vi "example_01.vi"() -> ()   [LabVIEW 2015, in "lv-recipe-machine.lvlib"]
uses:
  lv-recipe-machine.lvlib
  _controls/example_01_manual_actions.ctl
  public/_controls/step.ctl
  public/_controls/step_vi_reference.ctl
  public/_controls/mode.ctl
  _subvis/manual_test_comparison.vi
  _subvis/manual_test_wait.vi
  lv-recipe-machine_/repub-dvr_nre.lvlib
panel:
  out "data":variant
  in  "stop":bool
  in  "manual_action":T1=enum."test_random"
  in  "execute":bool
  in  "recipe":T2(ring)
  in  "resume":bool
  in  "abort":bool
  in  "pause":bool
  in  "start":bool
  in  "manual_mode":bool
  in  "automatic_mode":bool
  out "wait_elapsed_time":dbl format="%<%H:%M:%S>t"
  out "recipe_elapsed_time":dbl format="%<%H:%M:%S>t"
  out "random_data":dbl
  out "action":string
  out "state":string
  out "mode":string
  in  "events":i32(listbox)
  out "error out":errorcluster
  # "Manual Inputs"
  # "Automatic Inputs"
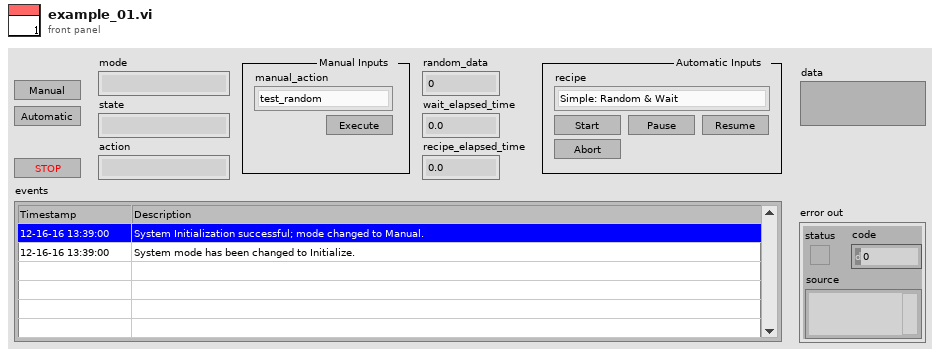
[diagram p1: front panel]
types:
  T1 = typedef "lv-recipe-machine.lvlib/example_01_manual_actions.ctl" = enum16{"<manual_action>", "test_random", "test_comparison", "test_wait", "<null>"}
  T2 = enum16{"Simple: Random & Wait", "Simple: Random & Test", "Intermediate: Fixed Continuous", "Intermediate: Test w/Continuous-Fail"}
  T3 = typedef "lv-recipe-machine.lvlib/step.ctl" = cluster{"name":string, "step_vi_reference":T4, "data":variant}
  T4 = typedef "lv-recipe-machine.lvlib/step_vi_reference.ctl" = refnum<vi>
  T5 = typedef "repub-dvr_nre.lvlib/references.ctl" = cluster{"semaphore":T6, "input_queue":refnum<queue>, "output_queue":refnum<queue>, "data_dvr":refnum<data-value>, "stop_notifier":refnum<notifier>, "transition_queue":refnum<queue>, "change_in_notifier":refnum<notifier>, "change_out_notifier":refnum<notifier>, "change_in_event":refnum<user-event>, "change_out_event":refnum<user-event>}
  T6 = typedef "Semaphore RefNum" = refnum<k1>
  T7 = typedef "lv-recipe-machine.lvlib/mode.ctl" = enum16{"<mode>", "manual", "automatic", "<null>"}
  T8 = typedef "repub-dvr_nre.lvlib/status.ctl" = cluster{"mode":T7, "manual_state":T9, "automatic_state":T10, "step":string}
  T9 = typedef "lv-recipe-machine.lvlib/manual_state.ctl" = enum16{"<manual_state>", "failed", "action", "running", "idle", "<null>"}
  T10 = typedef "lv-recipe-machine.lvlib/automatic_state.ctl" = enum16{"<automatic_state>", "failed", "idle", "running", "paused", "transition", "stopped", "<null>"}
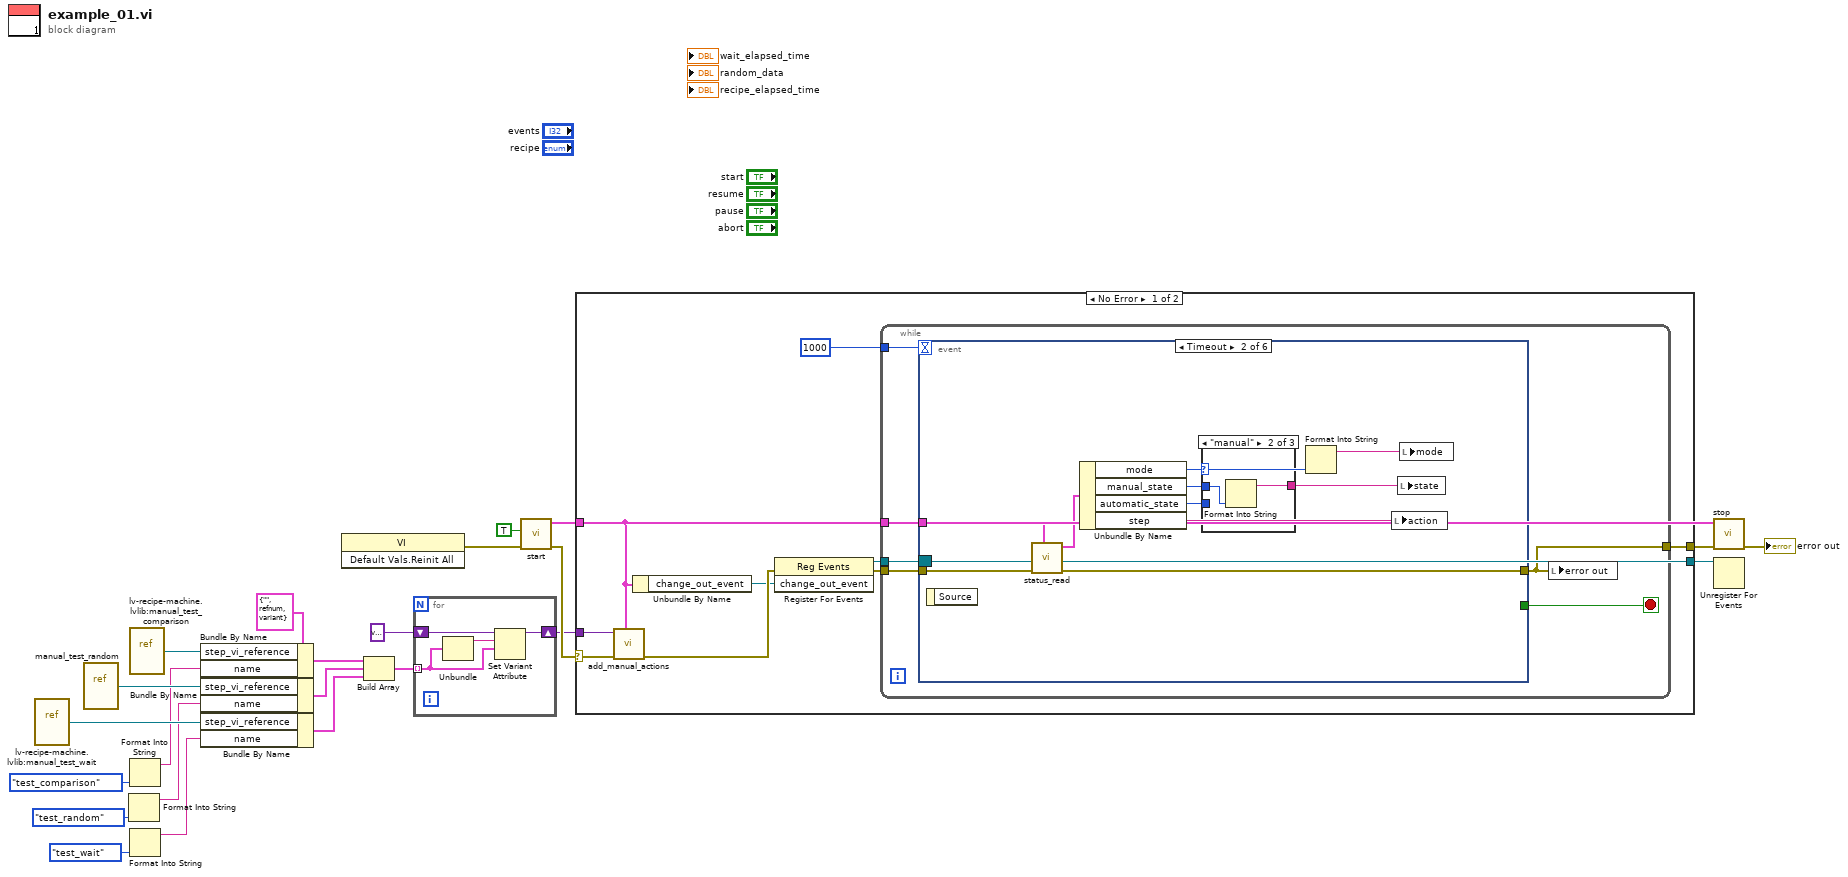
[diagram p0: block diagram]
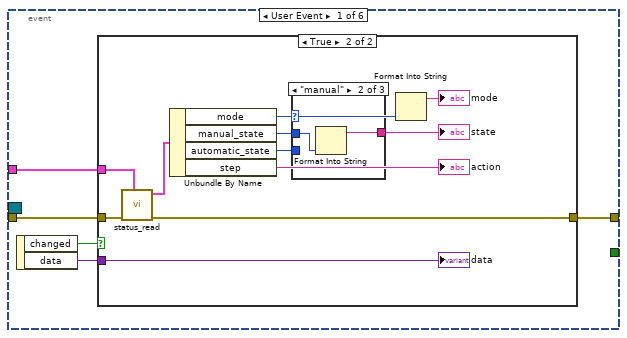
[diagram p2: hidden frame]
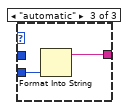
[diagram p5: hidden frame]
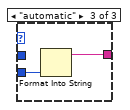
[diagram p7: hidden frame]
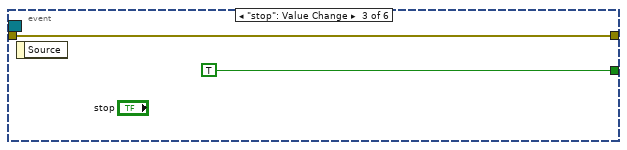
[diagram p8: hidden frame]
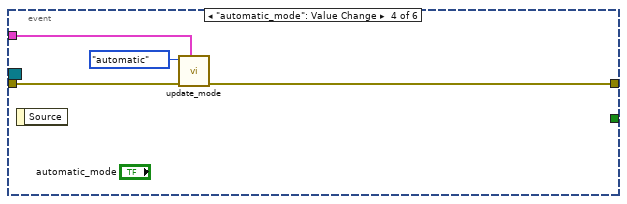
[diagram p9: hidden frame]
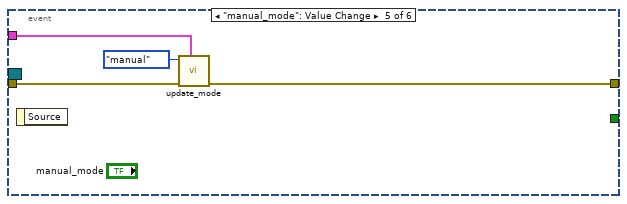
[diagram p10: hidden frame]
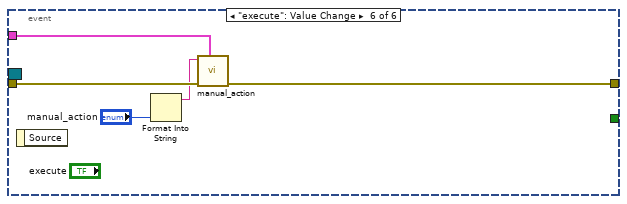
[diagram p11: hidden frame]
diagram:
  w9 = T3 {"name"="", "step_vi_reference"=refnum, "data"=variant} ("step")
  n1 = vi-ref "lv-recipe-machine.lvlib:manual_test_wait.vi"() -> (w4:refnum<vi>)
  n2 = vi-ref "manual_test_random.vi"() -> (w12:refnum<vi>)
  n3 = Format Into String(example_01_manual_actions."test_random" ("action")) -> (resulting string=w2:string)  [unwired: 3 in, 1 out]
  n4 = vi-ref "lv-recipe-machine.lvlib:manual_test_comparison.vi"() -> (w13:refnum<vi>)
  n5 = Format Into String(example_01_manual_actions."test_comparison" ("action")) -> (resulting string=w1:string)  [unwired: 3 in, 1 out]
  n6 = Format Into String(example_01_manual_actions."test_wait" ("action")) -> (resulting string=w3:string)  [unwired: 3 in, 1 out]
  n7 = Bundle By Name(cluster=w9, "step_vi_reference"=w13, "name"=w1) -> (w15:T3)
  n8 = Bundle By Name(cluster=w9, "step_vi_reference"=w12, "name"=w2) -> (w14:T3)
  n9 = Bundle By Name(cluster=w9, "step_vi_reference"=w4, "name"=w3) -> (w8:T3)
  n10 = invoke class="VI" method="Default Vals.Reinit All"() -> (error out=w22:errorcluster)  [unwired: 3 in, 2 out]
  n11 = Build Array(w15, w14, w8) -> (w11:T3[])
  n12 = for {
    tunnel: w11 -> [w25] mode=indexing
    shift-right: [w26] -> w10
    shift-left: variant ("recipe") -> [w27]
    n13 = Unbundle(w25) -> ("name"=w24:string)  [unwired: 2 out]
    n14 = Set Variant Attribute(Variant=w27, name=w24, value=w25) -> (Variant out=w26:variant)  [unwired: 1 in, 2 out]
  }
  n15 = call "start.vi"("error in (no error)"=w22, "enable_event"=TRUE) -> ("error out"=w21:errorcluster, "references"=w20:T5)  [unwired: 8 in]
  n16 = case shown="No Error" w21 {
    selector: w21 -> [w29 w93]
    tunnel: [w35 w93] -> w23
    tunnel: w20 -> [w31 _]
    tunnel: [w32 _] -> w18
    tunnel: w10 -> [w30 _]
    frame No Error {
      n17 = call "add_manual_actions.vi"("references"=w31, "error in (no error)"=w29, "manual_actions"=w30) -> ("error out"=w36:errorcluster)  [unwired: 8 in]
      n18 = Unbundle By Name(w31) -> ("change_out_event"=w33:refnum<user-event>)
      n19 = register-events(error in=w36, w33) -> (reference out=w32:refnum<event-registration>, error out=w34:errorcluster)  [unwired: 1 in]
      n20 = while {
        tunnel: w34 -> [w42]
        tunnel: [w38] -> w35
        tunnel: w31 -> [w40]
        tunnel: w32 -> [w39]
        tunnel: 1000 -> [w37]
        stop <- w41 stop-if-true
        n21 = event shown="[1] Timeout" {
          selector: w39 -> [_ _ _ _ _ _]
          dyn-events: _ -> [_ _ _ _ _ _]
          timeout: w37 -> [_ _ _ _ _ _]
          tunnel: w42 -> [w47 w73 w79 w82 w86 w92]
          tunnel: [w46 w72 w79 w83 w87 w89] -> w38
          tunnel: [_ _ TRUE _ _ _] -> w41
          tunnel: w40 -> [w45 w71 _ w81 w85 w88]
          event User Event {
            n22 = event-data() -> ("changed"=w44:bool, "data"=w43:variant)  [unwired: 1 in]
            n23 = case shown="True" w44 {
              tunnel: w47 -> [w48 w59]
              tunnel: [w48 w56] -> w46
              tunnel: w45 -> [_ w58]
              tunnel: w43 -> [_ w49]
              frame False {
              }
              frame True {
                n24 = call "status_read.vi"("references"=w58, "error in (no error)"=w59) -> ("error out"=w56:errorcluster, "status"=w57:T8)  [unwired: 8 in]
                n25 = Unbundle By Name(w57) -> ("mode"=w53:T7, "manual_state"=w55:T9, "automatic_state"=w54:T10, "step"=→"action":string)
                n26 = case shown="\"manual\"" w53 {
                  tunnel: w55 -> [_ w61 _]
                  tunnel: w54 -> [_ _ w62]
                  tunnel: [_ w60 w63] -> w51
                  frame Default {
                  }
                  frame "manual" {
                    n27 = Format Into String(w61) -> (resulting string=w60:string)  [unwired: 3 in, 1 out]
                  }
                  frame "automatic" {
                    n28 = Format Into String(w62) -> (resulting string=w63:string)  [unwired: 3 in, 1 out]
                  }
                }
                "state" <- w51
                n29 = Format Into String(w53) -> (resulting string=→"mode":string)  [unwired: 3 in, 1 out]
                "data" <- w49
              }
            }
          }
          event Timeout {
            n30 = event-data() -> ()  [unwired: 1 in, 1 out]
            n31 = call "status_read.vi"("references"=w71, "error in (no error)"=w73) -> ("error out"=w72:errorcluster, "status"=w70:T8)  [unwired: 8 in]
            n32 = Unbundle By Name(w70) -> ("mode"=w67:T7, "manual_state"=w69:T9, "automatic_state"=w68:T10, "step"=w64:string)
            n33 = case shown="\"manual\"" w67 {
              tunnel: w69 -> [_ w75 _]
              tunnel: w68 -> [_ _ w76]
              tunnel: [_ w74 w77] -> w65
              frame Default {
              }
              frame "manual" {
                n34 = Format Into String(w75) -> (resulting string=w74:string)  [unwired: 3 in, 1 out]
              }
              frame "automatic" {
                n35 = Format Into String(w76) -> (resulting string=w77:string)  [unwired: 3 in, 1 out]
              }
            }
            n36 = Format Into String(w67) -> (resulting string=w66:string)  [unwired: 3 in, 1 out]
            n37 = local write "action"(w64) -> ()
            n38 = local write "state"(w65) -> ()
            n39 = local write "mode"(w66) -> ()
          }
          event "stop": Value Change {
            n40 = event-data() -> ()  [unwired: 1 in, 1 out]
          }
          event "automatic_mode": Value Change {
            n41 = event-data() -> ()  [unwired: 1 in, 1 out]
            n42 = call "update_mode.vi"("references"=w81, "error in (no error)"=w82, "mode"=mode."automatic") -> ("error out"=w83:errorcluster)  [unwired: 8 in]
          }
          event "manual_mode": Value Change {
            n43 = event-data() -> ()  [unwired: 1 in, 1 out]
            n44 = call "update_mode.vi"("references"=w85, "error in (no error)"=w86, "mode"=mode."manual") -> ("error out"=w87:errorcluster)  [unwired: 8 in]
          }
          event "execute": Value Change {
            n45 = event-data() -> ()  [unwired: 1 in, 1 out]
            n46 = Format Into String("manual_action") -> (resulting string=w90:string)  [unwired: 3 in, 1 out]
            n47 = call "manual_action.vi"("references"=w88, "error in (no error)"=w92, "step"=w90) -> ("error out"=w89:errorcluster)  [unwired: 8 in]
          }
        }
        n48 = local write "error out"(w38) -> ()
      }
    }
    frame Error {
    }
  }
  n49 = call "stop.vi"("error in (no error)"=w23, "references"=w20) -> ("error out"=→"error out":errorcluster)  [unwired: 9 in]
  n50 = Unregister For Events(event registration refnum=w18) -> ()  [unwired: 1 in, 1 out]
